vi "FRC-Traj-Lib-analog-filter-test.vi"() -> ()   [LabVIEW 2019]
uses:
  <vilib>/Rock Robotics/WPI/ThirdParty/JAS_Junk/TrajLib/LINEAR_FILTER.ctl
  <vilib>/Rock Robotics/WPI/ThirdParty/JAS_Junk/TrajLib/LinearFilter_ResetToValue.vi
  <vilib>/Rock Robotics/WPI/ThirdParty/JAS_Junk/TrajLib/LinearFilter_Calculate.vi
  <vilib>/Rock Robotics/WPI/ThirdParty/JAS_Junk/TrajLib/LinearFilter_MovingAverage.vi
  <vilib>/Rock Robotics/WPI/ThirdParty/JAS_Junk/TrajLib/LinearFilter_LowPassBW1.vi
  <vilib>/Rock Robotics/WPI/ThirdParty/JAS_Junk/TrajLib/LinearFilter_LowPassBW2.vi
  <vilib>/Rock Robotics/WPI/ThirdParty/JAS_Junk/TrajLib/LinearFilter_HighPassBW1.vi
  <vilib>/Rock Robotics/WPI/ThirdParty/JAS_Junk/TrajLib/LinearFilter_HighPassBW2.vi
  <vilib>/Rock Robotics/WPI/ThirdParty/JAS_Junk/TrajLib/Trajectory_Library.lvlib
panel:
  in  "Auto / Manual":bool=TRUE
  in  "Noise":bool=TRUE
  in  "Filter Enable":bool=TRUE
  in  "Use White Noise":bool=TRUE
  in  "Tab Control 2":T1(tab)
  out "Avg3":cluster{dbl, dbl, "Value_Output":dbl}(graph)
  out "Avg3 Out Dial":dbl(knob)=-2.895988890827539e-05 scale=-20.0..20.0
  out "Avg3 Out":dbl format="%11.3f"
  out "Med3":cluster{dbl, dbl, "Value_Output":dbl}(graph)
  out "Med3 Out":dbl format="%11.3f"
  out "Med3 Out Dial":dbl(knob)=-2.895988890827539e-05 scale=-20.0..20.0
  out "Avg7":cluster{dbl, dbl, "Value_Output":dbl}(graph)
  out "Avg7 Out":dbl format="%11.3f"
  out "Avg7 Out Dial":dbl(knob)=-2.895988890827539e-05 scale=-20.0..20.0
  out "Med7":cluster{dbl, dbl, "Value_Output":dbl}(graph)
  out "Med7 Out":dbl format="%11.3f"
  out "Med7 Out Dial":dbl(knob)=-2.895988890827539e-05 scale=-20.0..20.0
  out "LP BW 2":cluster{dbl, dbl, "Output_Value":dbl}(graph)
  out "Butter 1 Out":dbl format="%11.3f"
  out "Low Pass Butterworth 1 Dial":dbl(knob)=-2.895988890827539e-05 scale=-20.0..20.0
  out "Fc 2":dbl format="%11.3f"
  out "BW1-FF-Consts":dbl[](array[numeric])
  out "BW1-FB-Consts":dbl[](array[numeric])
  out "LP BW 2":cluster{dbl, dbl, "Output_Value":dbl}(graph)
  out "Butter 2 Out":dbl format="%11.3f"
  out "Low Pass Butterworth 2 Dial":dbl(knob)=-2.895988890827539e-05 scale=-20.0..20.0
  out "Fc 3":dbl format="%11.3f"
  out "LP BW2 Cluster":T2 {"Outputs" format="%13.5g"; "Inputs" format="%13.5g"; "OutputGains" format="%13.5g"; "InputGains" format="%13.5g"}
  out "HP BW 1":cluster{dbl, dbl, "Output_Value":dbl}(graph)
  out "HP BW 1":dbl format="%11.3f"
  out "High Pass Butterworth 1":dbl(knob)=-2.895988890827539e-05 scale=-20.0..20.0
  out "HP  BW 2":cluster{dbl, dbl, "Output_Value":dbl}(graph)
  out "Alt Lag":dbl format="%11.3f"
  out "High Pass Butterworth 2":dbl(knob)=-2.895988890827539e-05 scale=-20.0..20.0
  out "Fc 1":dbl format="%11.3f"
  out "Duration":dbl format="%11.3f"
  out "Late":dbl format="%11.3f"
  in  "Manual\nInput":dbl(slide) min=-12.0 max=12.0 scale=-12.0..12.0
  out "Raw Noise":dbl(knob)=-2.895988890827539e-05 scale=-20.0..20.0
  out "Raw Noise":dbl format="%11.3f"
  out "Actual Input":dbl(knob)=-2.895988890827539e-05 scale=-20.0..20.0
  out "Actual Input":dbl format="%11.3f"
  in  "Time Const (Sec)":dbl=0.08 min=0.0 step=0.001 format="%10.4f"
  out "Input":cluster{"Manual\nInput":dbl, dbl, "f":dbl}(graph)
  out "Meas Dial":dbl(knob)=-2.895988890827539e-05 scale=-20.0..20.0
  out "Measured Value":dbl format="%11.3f"
  # "Example of Analog FIltering"
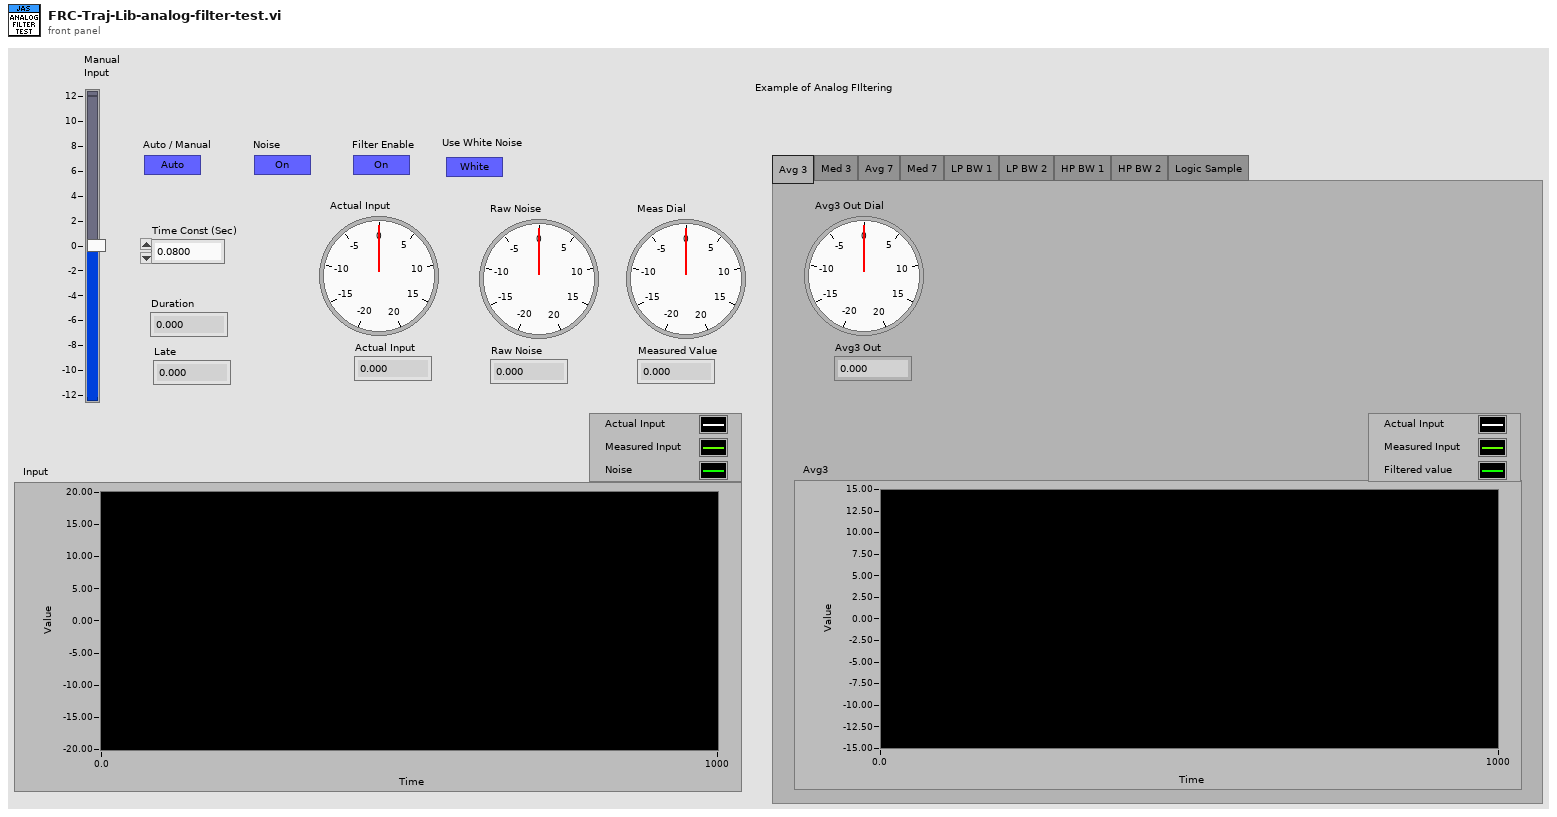
[diagram p1: front panel]
types:
  T1 = enum32{"Avg 3", "Med 3", "Avg 7", "Med 7", "LP BW 1", "LP BW 2", "HP BW 1", "HP BW 2", "Logic Sample"}
  T2 = typedef "Trajectory_Library.lvlib/LINEAR_FILTER.ctl" = cluster{"InputGains":dbl[], "OutputGains":dbl[], "Inputs":dbl[], "Outputs":dbl[], "InGainCount":i32, "OutGainCount":i32}
  T3 = enum16{"Moving Average", "Low Pass 1st Order Butterworth", "Low Pass 2nd Order Butterworth", "High Pass 1st Order Butterworth", "High Pass 2nd Order Butterworth"}
  T4 = cluster{"Manual\nInput":dbl, dbl, "MedianValue":dbl}
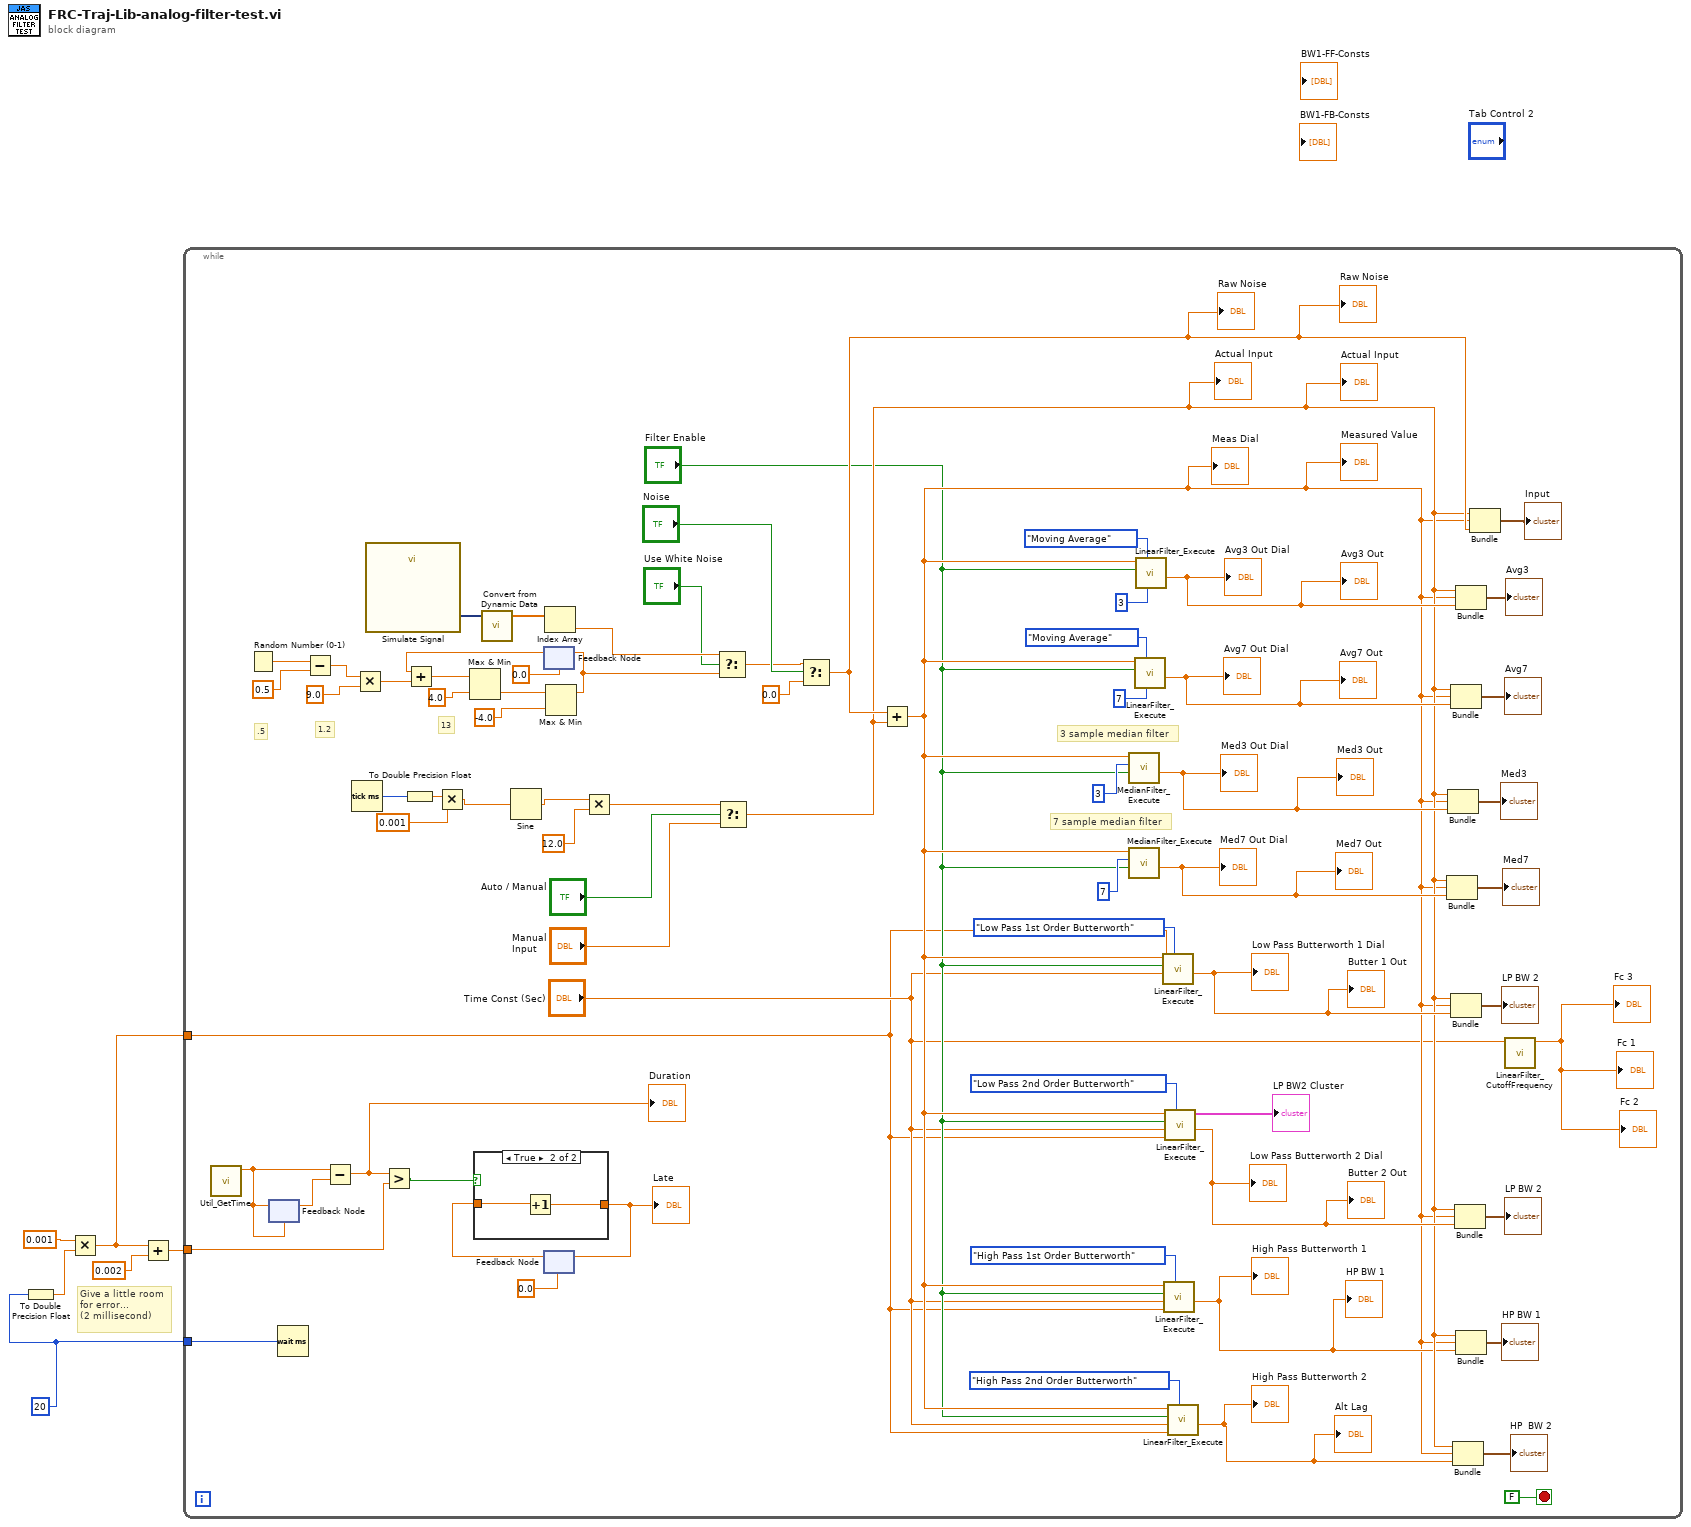
[diagram p0: block diagram]
diagram:
  w4 = u32 20 ("milliseconds to wait")
  # "Give a little room\nfor error...\n(2 millisecond)"
  n1 = To Double Precision Float(number=w4) -> (double precision float=w6:dbl)
  n2 = Multiply(x=0.001, y=w6) -> (x*y=w1:dbl)
  n3 = Add(x=w1, y=0.002) -> (x+y=w3:dbl)
  n4 = while {
    tunnel: w4 -> [w33]
    tunnel: w3 -> [w32]
    tunnel: w1 -> [w8]
    stop <- FALSE stop-if-true
    # "7 sample median filter"
    # "3 sample median filter"
    # "13"
    # "1.2"
    # ".5"
    n5 = call <vilib>:"Util_GetTime.vi"() -> ("FPGA_Time_Seconds"=w37:dbl)  [unwired: 10 in, 1 out]
    n6 = Random Number (0-1)() -> (number: 0 to 1=w74:dbl)
    n7 = feedback-in #1(w37) -> ()
    n8 = feedback #1(w37) -> (w36:dbl)
    n9 = Wait (ms)(milliseconds to wait=w33) -> ()  [unwired: 1 out]
    n10 = Subtract(x=w74, y=0.5) -> (x-y=w70:dbl)
    n11 = Subtract(x=w37, y=w36) -> (x-y=w34:dbl)
    "Duration" <- w34
    n12 = Tick Count (ms)() -> (millisecond timer value=w63:u32)
    n13 = Multiply(x=w70, y=9.0) -> (x*y=w69:dbl)
    n14 = call "Simulate Signal"() -> ("DC with Uniform Noise"=w51:dynamicdata)  [unwired: 14 in, 1 out]
    n15 = Greater?(x=w34, y=w32) -> (0:w35:bool)
    n16 = To Double Precision Float(number=w63) -> (double precision float=w64:dbl)
    n17 = Multiply(x=w64, y=0.001) -> (x*y=w61:dbl)
    n18 = call "Convert from Dynamic Data"("Dynamic Data Type"=w51) -> ("Array"=w50:dbl[])  [unwired: 3 in]
    n19 = Sine(x=w61) -> (sin(x)=w60:dbl)
    n20 = feedback #2(0.0) -> (w71:dbl)
    n21 = Add(x=w71, y=w69) -> (x+y=w73:dbl)
    n22 = Max & Min(x=w73, y=4.0) -> (min(x,y)=w72:dbl)  [unwired: 1 out]
    n23 = feedback #3(0.0) -> (w44:dbl)
    n24 = case shown="True" w35 {
      tunnel: [w80 w82] -> w45
      tunnel: w44 -> [w80 w81]
      frame False {
      }
      frame True {
        n25 = Increment(x=w81) -> (x+1=w82:dbl)
      }
    }
    "Late" <- w45
    n26 = feedback-in #3(w45) -> ()
    n27 = Index Array(array=w50) -> (element=w49:dbl)  [unwired: 1 in]
    n28 = Max & Min(x=w72, y=-4.0) -> (max(x,y)=w52:dbl)  [unwired: 1 out]
    n29 = feedback-in #2(w52) -> ()
    n30 = Multiply(x=w60, y=12.0) -> (x*y=w57:dbl)
    n31 = Select(t=w49, s="Use White Noise", f=w52) -> (s? t:f=w53:dbl)
    n32 = Select(t=w57, s="Auto / Manual", f="Manual\nInput") -> (s? t:f=w16:dbl)
    "Actual Input" <- w16
    "Actual Input" <- w16
    n33 = Select(t=w53, s="Noise", f=0.0) -> (s? t:f=w47:dbl)
    "Raw Noise" <- w47
    "Raw Noise" <- w47
    n34 = Add(x=w47, y=w16) -> (x+y=w11:dbl)
    "Measured Value" <- w11
    "Meas Dial" <- w11
    n35 = call <vilib>:"MedianFilter_Execute.vi"("Enable"="Filter Enable", "Samples"=3, "Input Value"=w11) -> ("MedianValue"=w28:dbl)  [unwired: 7 in, 1 out]
    "Med3 Out" <- w28
    "Med3 Out Dial" <- w28
    n36 = call <vilib>:"MedianFilter_Execute.vi"("Enable"="Filter Enable", "Samples"=7, "Input Value"=w11) -> ("MedianValue"=w30:dbl)  [unwired: 7 in, 1 out]
    "Med7 Out" <- w30
    "Med7 Out Dial" <- w30
    n37 = call <vilib>:"LinearFilter_Execute.vi"("Samples"=7, "Filter Type"=T3."Moving Average", "Enable"="Filter Enable", "Input"=w11) -> ("Output"=w39:dbl)  [unwired: 6 in, 1 out]
    "Avg7 Out" <- w39
    "Avg7 Out Dial" <- w39
    n38 = call <vilib>:"LinearFilter_Execute.vi"("Samples"=3, "Filter Type"=T3."Moving Average", "Enable"="Filter Enable", "Input"=w11) -> ("Output"=w40:dbl)  [unwired: 6 in, 1 out]
    "Avg3 Out" <- w40
    "Avg3 Out Dial" <- w40
    n39 = call <vilib>:"LinearFilter_Execute.vi"("Filter Type"=T3."Low Pass 1st Order Butterworth", "SamplePeriod"=w8, "TimeConstant"="Time Const (Sec)", "Enable"="Filter Enable", "Input"=w11) -> ("Output"=w31:dbl)  [unwired: 5 in, 1 out]
    "Butter 1 Out" <- w31
    "Low Pass Butterworth 1 Dial" <- w31
    n40 = call <vilib>:"LinearFilter_Execute.vi"("Filter Type"=T3."High Pass 1st Order Butterworth", "SamplePeriod"=w8, "TimeConstant"="Time Const (Sec)", "Enable"="Filter Enable", "Input"=w11) -> ("Output"=w12:dbl)  [unwired: 5 in, 1 out]
    "High Pass Butterworth 1" <- w12
    "HP BW 1" <- w12
    n41 = call <vilib>:"LinearFilter_Execute.vi"("Filter Type"=T3."Low Pass 2nd Order Butterworth", "SamplePeriod"=w8, "TimeConstant"="Time Const (Sec)", "Enable"="Filter Enable", "Input"=w11) -> ("Output"=w19:dbl, "Out LINEAR_FILTER"=→"LP BW2 Cluster":T2)  [unwired: 5 in]
    "Butter 2 Out" <- w19
    "Low Pass Butterworth 2 Dial" <- w19
    n42 = call <vilib>:"LinearFilter_Execute.vi"("Filter Type"=T3."High Pass 2nd Order Butterworth", "SamplePeriod"=w8, "TimeConstant"="Time Const (Sec)", "Enable"="Filter Enable", "Input"=w11) -> ("Output"=w13:dbl)  [unwired: 5 in, 1 out]
    "Alt Lag" <- w13
    "High Pass Butterworth 2" <- w13
    n43 = Bundle("Manual\nInput"=w16, w11, "MedianValue"=w30) -> (→"Med7":T4)  [unwired: 1 in]
    n44 = Bundle("Manual\nInput"=w16, w11, "MedianValue"=w28) -> (→"Med3":T4)  [unwired: 1 in]
    n45 = Bundle("Manual\nInput"=w16, w11, "Output"=w39) -> (→"Avg7":cluster{"Manual\nInput":dbl, dbl, "Output":dbl})  [unwired: 1 in]
    n46 = Bundle("Manual\nInput"=w16, w11, "Output"=w31) -> (→"LP BW 2":cluster{"Manual\nInput":dbl, dbl, "Output":dbl})  [unwired: 1 in]
    n47 = Bundle("Manual\nInput"=w16, w11, "Output"=w13) -> (→"HP  BW 2":cluster{"Manual\nInput":dbl, dbl, "Output":dbl})  [unwired: 1 in]
    n48 = Bundle("Manual\nInput"=w16, w11, "Output"=w19) -> (→"LP BW 2":cluster{"Manual\nInput":dbl, dbl, "Output":dbl})  [unwired: 1 in]
    n49 = Bundle("Manual\nInput"=w16, w11, "Output"=w40) -> (→"Avg3":cluster{"Manual\nInput":dbl, dbl, "Output":dbl})  [unwired: 1 in]
    n50 = Bundle("Manual\nInput"=w16, w11, "Output"=w12) -> (→"HP BW 1":cluster{"Manual\nInput":dbl, dbl, "Output":dbl})  [unwired: 1 in]
    n51 = Bundle("Manual\nInput"=w16, w11, "f"=w47) -> (→"Input":cluster{"Manual\nInput":dbl, dbl, "f":dbl})  [unwired: 1 in]
    n52 = call <vilib>:"LinearFilter_CutoffFrequency.vi"("TimeConstant"="Time Const (Sec)") -> ("Cutoff Freq"=→"Fc 1" →"Fc 2" →"Fc 3":dbl)  [unwired: 10 in]
  }
